vi "Unit Test.vi"() -> ()   [LabVIEW 2018]
uses:
  PPLs/Digital Delay Generator/Parent/Digital Delay Generator.lvlibp/Custom Controls/Trigger Mode.ctl
  PPLs/Digital Delay Generator/Parent/Digital Delay Generator.lvlibp/Custom Controls/Channel.ctl
  DG645.lvclass
  PPLs/Digital Delay Generator/Parent/Digital Delay Generator.lvlibp/Digital Delay Generator.lvclass
  C:/Projects/LabVIEW/PPLs/Digital Delay Generator/Parent/Digital Delay Generator.lvlibp/Digital Delay Generator.lvclass
panel:
  out "Connected":bool
  in  "Polarity (Positive:T)":bool=TRUE
  in  "Amplitude":dbl
  in  "Offset":dbl
  in  "Channel 2":T1
  in  "Channel 1":T1
  in  "Link Ch":bool
  in  "Delay (s)":dbl format="%#_6e"
  in  "Reference Channel":T1
  in  "Target Channel":T1
  in  "Level (V)":dbl
  in  "Trigger Rate (MHz)":dbl format="%#_13e"
  in  "Trigger Mode":T2
  in  "Configure":bool
  in  "Device Resource":string="TCPIP0::192.168.0.200::inst0::INSTR"
  in  "Reset":bool
  out "Status":string
  in  "Self Test":bool
  in  "Stop Button":bool
  # "Settings"
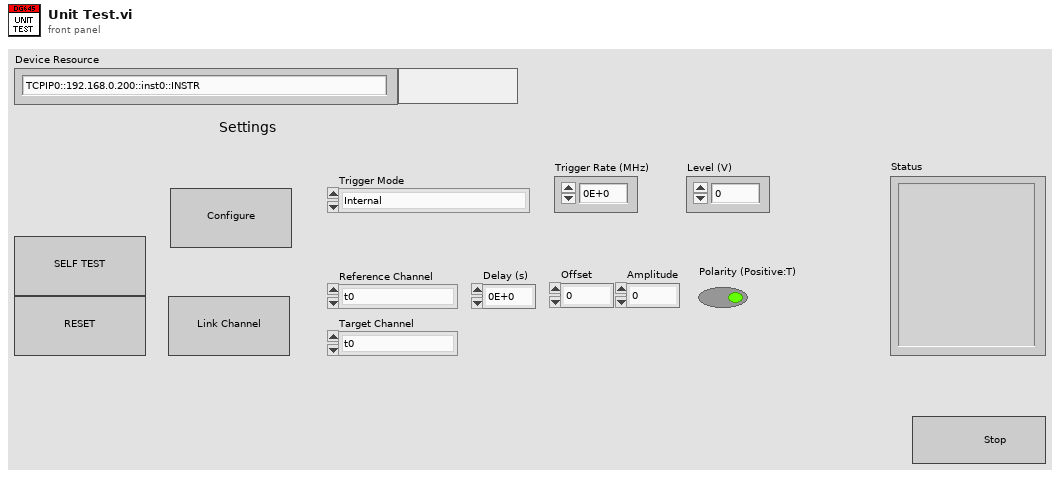
[diagram p1: front panel]
types:
  T1 = typedef "Digital Delay Generator.lvlibp/Digital Delay Generator.lvclass/Channel.ctl" = enum16{"t0", "A", "B", "C", "D", "E", "F", "G", "H"}
  T2 = typedef "Digital Delay Generator.lvlibp/Digital Delay Generator.lvclass/Trigger Mode.ctl" = enum16{"Internal", "External Rising Edge", "External Falling Edge", "Single Shot Internal Rising Edge", "Single Shot External Rising Edge", "Single Shot", "Line"}
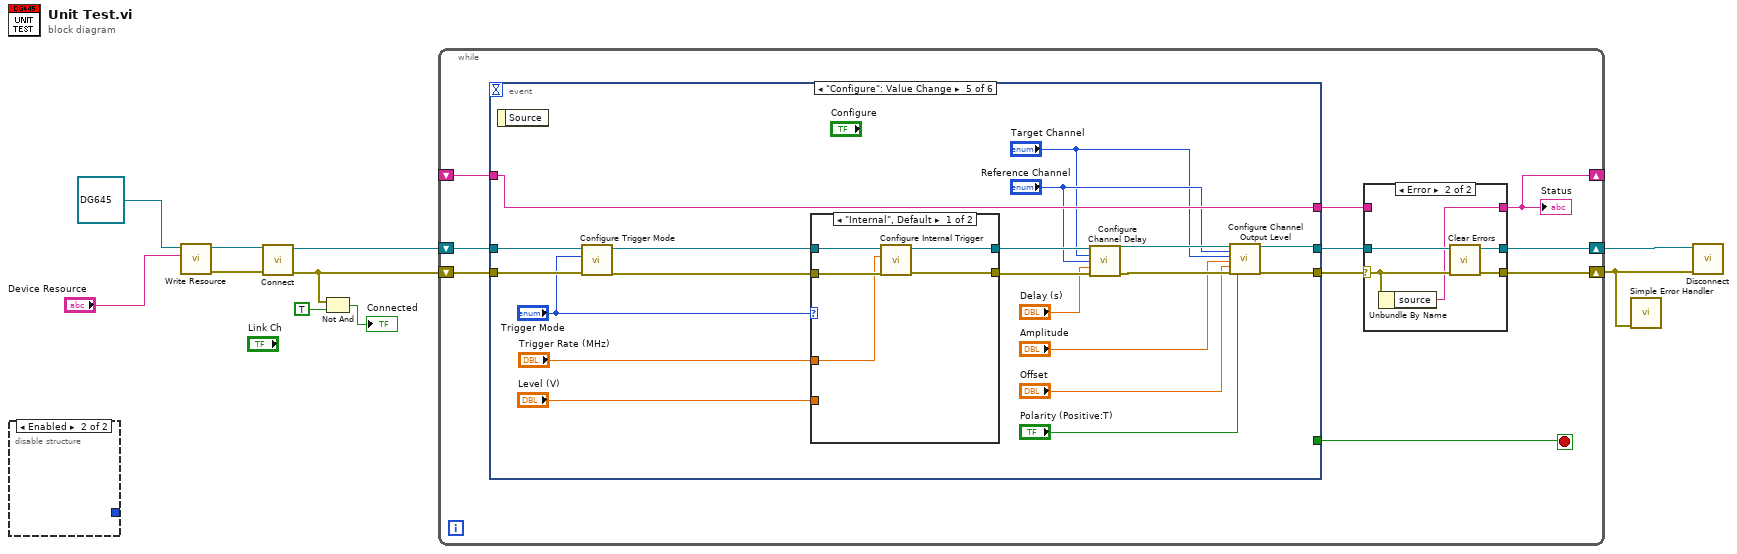
[diagram p0: block diagram]
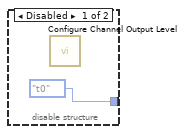
[diagram p2: hidden frame]
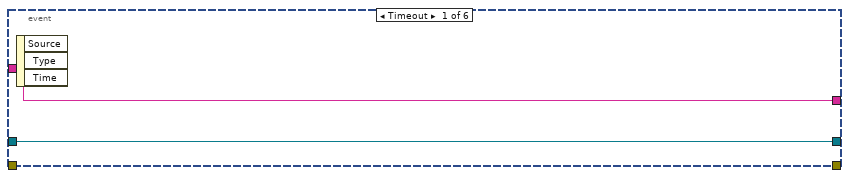
[diagram p4: hidden frame]
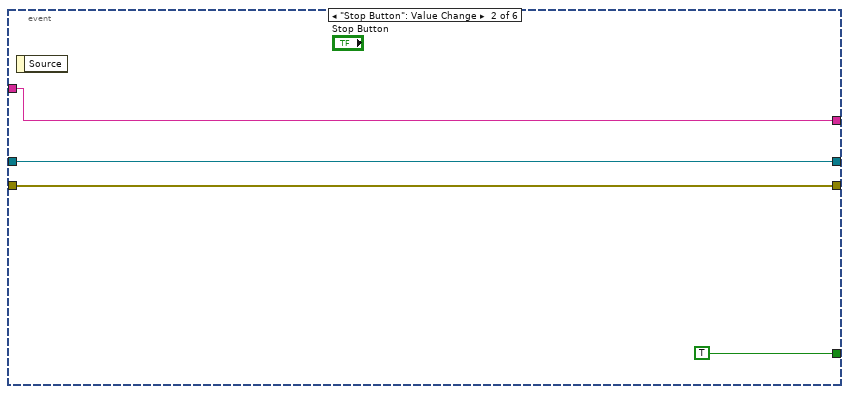
[diagram p5: hidden frame]
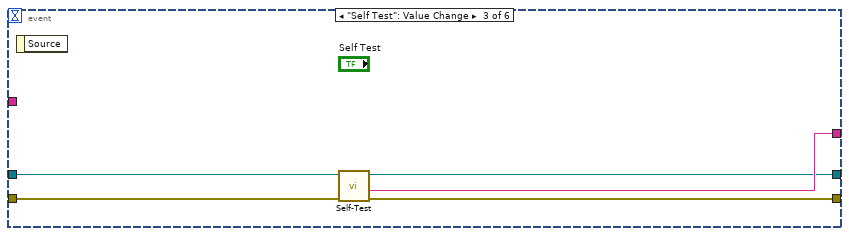
[diagram p6: hidden frame]
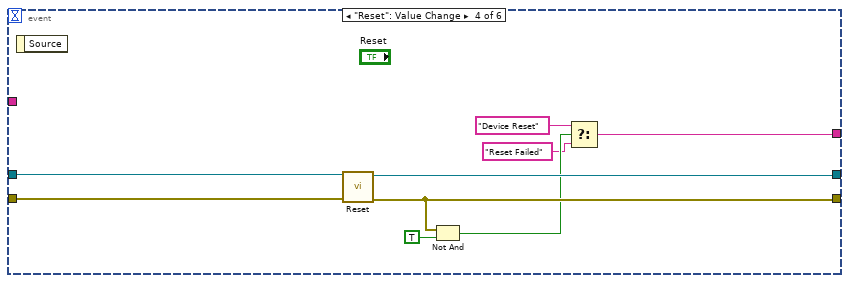
[diagram p7: hidden frame]
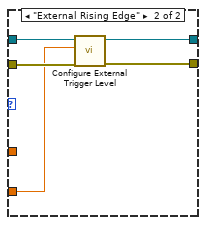
[diagram p8: hidden frame]
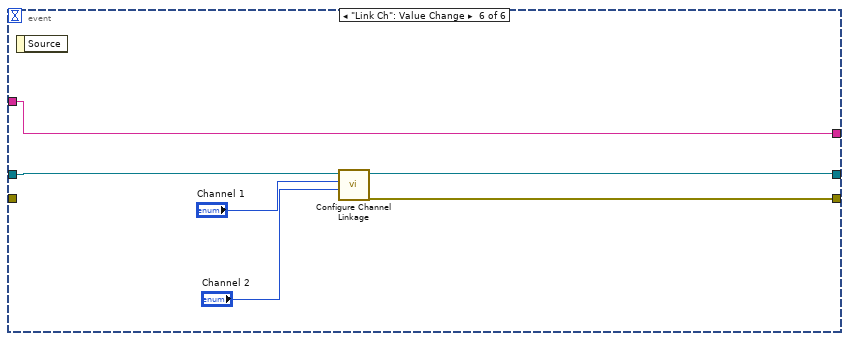
[diagram p9: hidden frame]
diagram:
  n1 = disable-structure shown="Enabled" {
    disable-tunnel: [Channel."t0" ("Channel 1") _] -> _
    frame Disabled {
      n2 = call-dynamic "Configure Channel Output Level.vi"() -> ()  [unwired: 18 in, 2 out]
    }
    frame Enabled {
    }
  }
  n3 = call "Write Resource.vi"("Resource"="Device Resource", "Digital Delay Generator in"=refnum<class "DG645.lvclass"> refnum ("DG645.lvlib:DG645.lvclass")) -> ("error out"=w8:errorcluster, "Digital Delay Generator out"=w9:refnum<class "DG645.lvclass">)  [unwired: 8 in]
  n4 = call-dynamic "Connect.vi"("error in (no error)"=w8, "DG645 in"=w9) -> ("error out"=w2:errorcluster, "DG645 out"=w7:refnum<class "DG645.lvclass">)  [unwired: 8 in]
  n5 = Not And(1:TRUE ("y"), 2:w2) -> (0:→"Connected":bool)
  n6 = while {
    shift-right: [w14] -> w6
    shift-left: w7 -> [w20]
    shift-right: [w16] -> w5
    shift-left: w2 -> [w19]
    shift-right: [w12] -> _
    shift-left: _ -> [w18]
    stop <- w21 stop-if-true
    n7 = event shown="[4] \"Configure\": Value Change" {
      selector: _ -> [_ _ _ _ _ _]
      dyn-events: _ -> [_ _ _ _ _ _]
      timeout: _ -> [_ _ _ _ _ _]
      tunnel: [_ TRUE _ _ _ _] -> w21
      tunnel: w20 -> [w29 w33 w39 w48 w66 w83]
      tunnel: w19 -> [_ w31 w38 w46 w67 _]
      tunnel: [w30 w32 w37 w41 w68 w84] -> w13
      tunnel: w18 -> [w30 w32 _ _ w68 w84]
      tunnel: [_ w31 w36 w44 w55 w81] -> w17
      tunnel: [w29 w33 w35 w47 w54 w82] -> w15
      event Timeout {
        n8 = event-data() -> ()  [unwired: 1 in, 3 out]
      }
      event "Stop Button": Value Change {
        n9 = event-data() -> ()  [unwired: 1 in, 1 out]
      }
      event "Self Test": Value Change {
        n10 = event-data() -> ()  [unwired: 1 in, 1 out]
        n11 = call-dynamic "Self-Test.vi"("error in (no error)"=w38, "DG645 in"=w39) -> ("error out"=w36:errorcluster, "Result Message"=w37:string, "DG645 out"=w35:refnum<class "DG645.lvclass">)  [unwired: 6 in, 1 out]
      }
      event "Reset": Value Change {
        n12 = event-data() -> ()  [unwired: 1 in, 1 out]
        n13 = call-dynamic "Reset.vi"("error in (no error)"=w46, "DG645 in"=w48) -> ("error out"=w44:errorcluster, "DG645 out"=w47:refnum<class "DG645.lvclass">)  [unwired: 8 in]
        n14 = Not And(1:TRUE ("y"), 2:w44) -> (0:w43:bool)
        n15 = Select(t="Device Reset" ("source"), s=w43, f="Reset Failed" ("source")) -> (s? t:f=w41:string)
      }
      event "Configure": Value Change {
        n16 = event-data() -> ()  [unwired: 1 in, 1 out]
        n17 = call-dynamic "Configure Trigger Mode.vi"("error in (no error)"=w67, "Trigger Mode"="Trigger Mode", "DG645 in"=w66) -> ("error out"=w61:errorcluster, "DG645 out"=w62:refnum<class "DG645.lvclass">)  [unwired: 7 in]
        n18 = case shown="\"Internal\", Default" "Trigger Mode" {
          tunnel: w62 -> [w73 w78]
          tunnel: w61 -> [w72 w76]
          tunnel: [w71 w75] -> w59
          tunnel: [w70 w77] -> w60
          tunnel: "Trigger Rate (MHz)" -> [w69 _]
          tunnel: "Level (V)" -> [_ w74]
          frame "Internal", Default {
            n19 = call-dynamic "Configure Internal Trigger.vi"("error in (no error)"=w72, "Internal Trigger Rate (1 MHz)"=w69, "DG645 in"=w73) -> ("error out"=w71:errorcluster, "DG645 out"=w70:refnum<class "DG645.lvclass">)  [unwired: 7 in]
          }
          frame "External Rising Edge" {
            n20 = call-dynamic "Configure External Trigger Level.vi"("error in (no error)"=w76, "Level (V)"=w74, "DG645 in"=w78) -> ("error out"=w75:errorcluster, "DG645 out"=w77:refnum<class "DG645.lvclass">)  [unwired: 7 in]
          }
        }
        n21 = call-dynamic "Configure Channel Delay.vi"("DG645 in"=w60, "Target Channel"="Target Channel", "Reference Channel"="Reference Channel", "Delay (s)"="Delay (s)", "error in (no error)"=w59) -> ("DG645 out"=w56:refnum<class "DG645.lvclass">, "error out"=w57:errorcluster)  [unwired: 9 in]
        n22 = call-dynamic "Configure Channel Output Level.vi"("DG645 in"=w56, "Rising Channel"="Reference Channel", "Falling Channel"="Target Channel", "Amplitude"="Amplitude", "Offset"="Offset", "error in (no error)"=w57, "Polarity (Positive:T)"="Polarity (Positive:T)") -> ("DG645 out"=w54:refnum<class "DG645.lvclass">, "error out"=w55:errorcluster)  [unwired: 11 in]
      }
      event "Link Ch": Value Change {
        n23 = event-data() -> ()  [unwired: 1 in, 1 out]
        n24 = call-dynamic "Configure Channel Linkage.vi"("Channel 2"="Channel 2", "Channel 1"="Channel 1", "DG645 in"=w83) -> ("error out"=w81:errorcluster, "DG645 out"=w82:refnum<class "DG645.lvclass">)  [unwired: 7 in]
      }
    }
    n25 = case shown="Error" w17 {
      selector: w17 -> [w23 w28]
      tunnel: [w23 w27] -> w16
      tunnel: w15 -> [w24 w26]
      tunnel: [w24 w26] -> w14
      tunnel: w13 -> [w22 _]
      tunnel: [w22 w25] -> w12
      frame No Error {
      }
      frame Error {
        n26 = Unbundle By Name(w28) -> ("source"=w25:string)
        n27 = call <vilib>:"Clear Errors.vi"("error in (no error)"=w28) -> ("error out"=w27:errorcluster)  [unwired: 5 in, 1 out]
      }
    }
    "Status" <- w12
  }
  n28 = call <vilib>:"Simple Error Handler.vi"("error in (no error)"=w5) -> ()  [unwired: 4 in, 5 out]
  n29 = call-dynamic "Disconnect.vi"("error in (no error)"=w5, "DG645 in"=w6) -> ()  [unwired: 8 in, 2 out]
